vi "MJG_XYZStageOffsets.vi"() -> ()   [LabVIEW 2016]
panel:
  out "XYZ Offsets [enc cnts]":i32[](array[numeric])
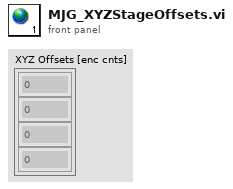
[diagram p1: front panel]
diagram:
